vi "Waveform Attribute, Set DBL Reference Array.vi"(5 "Refnum Array":refnum<vi>[](array[refnum]), 6 "error in":errorcluster, 9 "waveform":waveform(dbl)) -> (0 "error out":errorcluster, 3 "waveform out":waveform(dbl))   [LabVIEW 2010]
doc: "Writes a array of Digital double precision (DBL) values as waveform attributes using a control references."
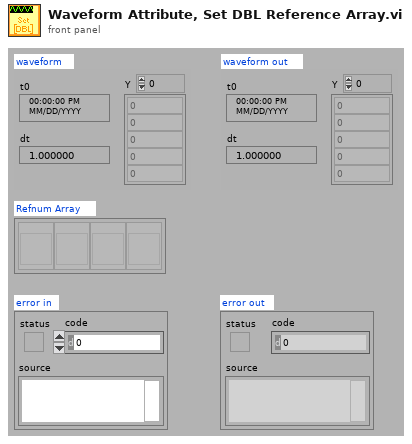
[diagram p1: front panel]
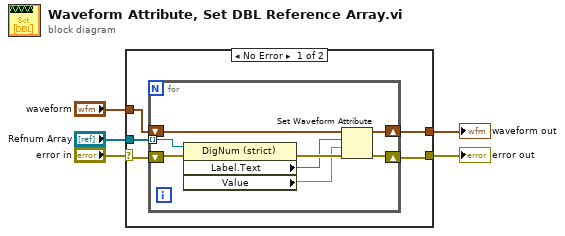
[diagram p0: block diagram]
diagram:
  n1 = case shown="No Error" "error in" {
    selector: "error in" -> [w8 w20]
    tunnel: [w9 w20] -> w5
    tunnel: "waveform" -> [w7 w19]
    tunnel: "Refnum Array" -> [w10 _]
    tunnel: [w6 w19] -> w1
    frame No Error {
      n2 = for {
        tunnel: w10 -> [w15] mode=indexing
        shift-right: [w14] -> w9
        shift-left: w8 -> [w13]
        shift-right: [w11] -> w6
        shift-left: w7 -> [w12]
        n3 = property class="DigNum (strict)"(reference=w15, error in=w13) -> (error out=w18:errorcluster, "Label.Text"=w16:string, "Value"=w17:dbl)  [unwired: 1 out]
        n4 = Set Waveform Attribute(4:w18, 5:w17, 6:w16, 7:w12) -> (0:w14:errorcluster, 3:w11:waveform(dbl))  [unwired: 1 out]
      }
    }
    frame Error {
    }
  }
  "error out" <- w5
  "waveform out" <- w1
